vi "WPI_RobotDriveRefNum Registry Get.vi"(10 "refnum name":string) -> (3 "RobotDriveDevRef":string)   [LabVIEW 2017]
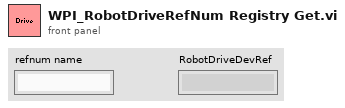
[diagram p1: front panel]
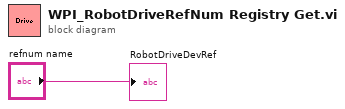
[diagram p0: block diagram]
diagram:
  "RobotDriveDevRef" <- "refnum name"
